vi "String Name.vi"() -> (4 "string name":string="niDCPower")   [LabVIEW 2021, in "Converter Reusables.lvlib"]
uses:
  Converter Reusables.lvlib
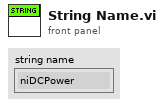
[diagram p1: front panel]
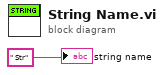
[diagram p0: block diagram]
diagram:
  "string name" <- " Str" ("Pin Name")
